vi "Buffer Assignments.vi"(9 "data string":string, 10 "Operation":enum16{"Append", "Retrieve"}(ring), 11 "TCP Network Connection in":refnum<k5>) -> (1 "TCP Data":string)   [LabVIEW 2017]
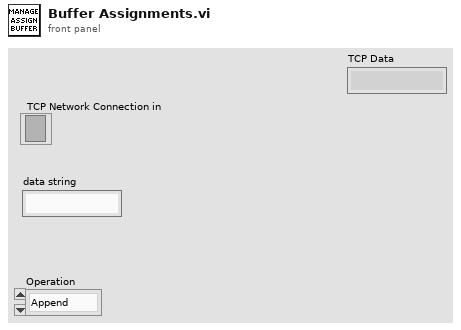
[diagram p1: front panel]
types:
  T1 = cluster{"TCP Network Connection in":refnum<k5>, "data string":string}[]
  T2 = cluster{"TCP Network Connection in":refnum<k5>, "data string":string}
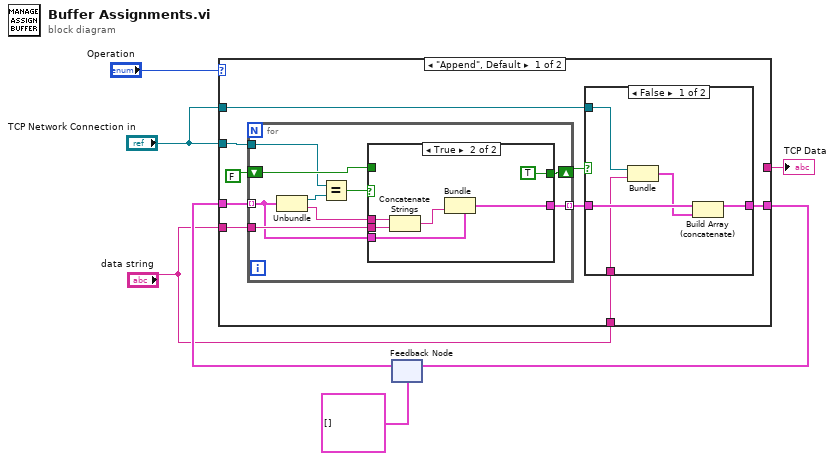
[diagram p0: block diagram]
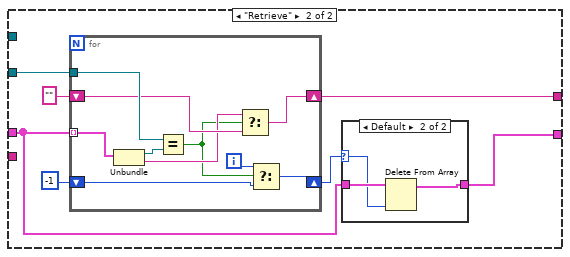
[diagram p4: hidden frame]
diagram:
  n1 = feedback #1(T1 []) -> (w6:T1)
  n2 = case shown="\"Append\", Default" "Operation" {
    tunnel: "TCP Network Connection in" -> [w16 w46]
    tunnel: w6 -> [w15 w41]
    tunnel: "data string" -> [w14 _]
    tunnel: [w11 w40] -> w5
    tunnel: "data string" -> [w9 _]
    tunnel: "TCP Network Connection in" -> [w8 _]
    tunnel: [_ w44] -> w1
    frame "Append", Default {
      n3 = for {
        tunnel: w16 -> [w23]
        tunnel: w15 -> [w28] mode=indexing
        tunnel: w14 -> [w29]
        tunnel: [w27] -> w10 mode=indexing
        shift-right: [w25] -> w12
        shift-left: FALSE -> [w24]
        n4 = Unbundle(w28) -> ("TCP Network Connection in"=w31:refnum<k5>, "data string"=w30:string)
        n5 = Equal?(x=w23, y=w31) -> (x = y?=w26:bool)
        n6 = case shown="True" w26 {
          tunnel: w30 -> [_ w39]
          tunnel: w29 -> [_ w38]
          tunnel: w28 -> [w32 w37]
          tunnel: [w32 w35] -> w27
          tunnel: [w33 TRUE] -> w25
          tunnel: w24 -> [w33 _]
          frame False {
          }
          frame True {
            n7 = Concatenate Strings(w39, w38) -> (w36:string)
            n8 = Bundle(cluster=w37, "data string"=w36) -> (w35:T2)  [unwired: 1 in]
          }
        }
      }
      n9 = case shown="False" w12 {
        tunnel: [w20 w22] -> w11
        tunnel: w10 -> [w21 w22]
        tunnel: w8 -> [w19 _]
        tunnel: w9 -> [w18 _]
        frame False {
          n10 = Bundle("TCP Network Connection in"=w19, "data string"=w18) -> (w17:T2)  [unwired: 1 in]
          n11 = Build Array (concatenate)(w21, w17) -> (w20:T1)
        }
        frame True {
        }
      }
    }
    frame "Retrieve" {
      n12 = for {
        tunnel: w41 -> [w59] mode=indexing
        tunnel: w46 -> [w58]
        shift-right: [w56] -> w44
        shift-left: "" ("data string") -> [w57]
        shift-right: [w51] -> w42
        shift-left: -1 -> [w52]
        i -> [w53]
        n13 = Unbundle(w59) -> ("TCP Network Connection in"=w60:refnum<k5>, "data string"=w55:string)
        n14 = Equal?(x=w58, y=w60) -> (x = y?=w54:bool)
        n15 = Select(t=w55, s=w54, f=w57) -> (s? t:f=w56:string)
        n16 = Select(t=w53, s=w54, f=w52) -> (s? t:f=w51:i32)
      }
      n17 = case shown="Default" w42 {
        selector: w42 -> [_ w48]
        tunnel: w41 -> [w47 w50]
        tunnel: [w47 w49] -> w40
        frame -1 {
        }
        frame Default {
          n18 = Delete From Array(array=w50, index=w48) -> (array with subset deleted=w49:T1)  [unwired: 1 in, 1 out]
        }
      }
    }
  }
  "TCP Data" <- w1
  n19 = feedback-in #1(w5) -> ()
